vi "Get_pixel_ptr.vi"(0 "Image In":T2) -> (1 "Image Out":T2, 2 "output cluster":T1)   [LabVIEW 2010]
uses:
  <vilib>/vision/Image Controls.llb/IMAQ Image.ctl
  Program Files/National Instruments/LabVIEW 2010/resource/objmgr/IMAQImage.rc
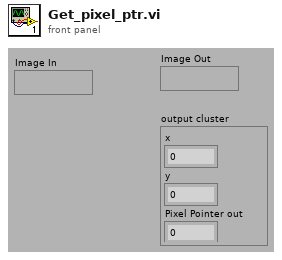
[diagram p1: front panel]
types:
  T1 = cluster{"x":i32, "y":i32, "Pixel Pointer out":u32}
  T2 = typedef "IMAQ Image.ctl" = refnum<image>
  T3 = enum32{"Map Pixel Pointer", "Unmap Pixel Pointer", "Get Pixels Infos"}
  T4 = cluster{"x":i32, "y":i32, "Pixel Pointer out":u64}
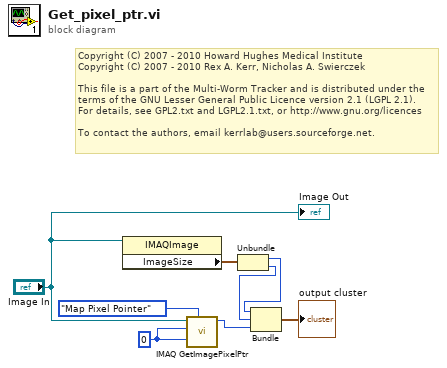
[diagram p0: block diagram]
diagram:
  w6 = 0 ("X Coordinate")
  # "Copyright (C) 2007 - 2010 Howard Hughes Medical Institute\nCopyright (C) 2007 - 2010 Rex A. Kerr, Nicholas A. Swierczek\n \nThis file is a part of the Multi-Worm Tracker and is distributed under the\nterms of the GNU Lesser General Public Licence version 2.1 (LGPL 2.1).\nFor details, see GPL2.txt and LGPL2.1.txt, or http://www.gnu.org/licences\n \nTo contact the authors, email kerrlab@users.sourceforge.net."
  n1 = property class="IMAQImage"(reference="Image In") -> ("ImageSize"=w7:cluster{"x":i32, "y":i32})  [unwired: 1 in, 2 out]
  n2 = call "IMAQ GetImagePixelPtr"("Function"=T3."Map Pixel Pointer", "Y Coordinate"=w6, "X Coordinate"=w6, "Image"="Image In") -> ("Pixel Pointer out"=w5:u64)  [unwired: 2 in, 5 out]
  n3 = Unbundle(w7) -> ("x"=w4:i32, "y"=w3:i32)
  n4 = Bundle("x"=w4, "y"=w3, "Pixel Pointer out"=w5) -> (→"output cluster":T4)  [unwired: 1 in]
  "Image Out" <- "Image In"
